vi "Corresponding Answer (SubVI).vi"(1 "Command":string, 2 "Tracker Response":string) -> (8 "Boolean":bool)   [LabVIEW 2017]
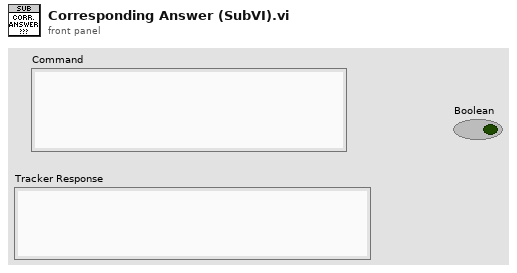
[diagram p1: front panel]
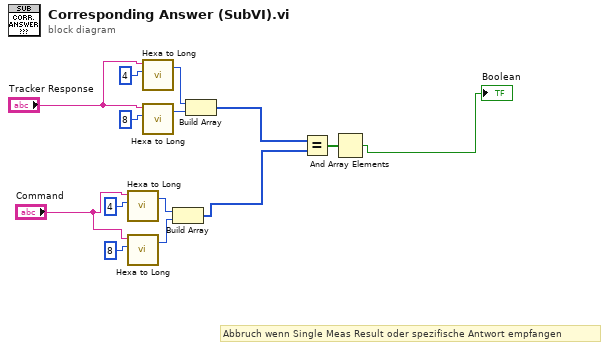
[diagram p0: block diagram]
diagram:
  # "Abbruch wenn Single Meas Result oder spezifische Antwort empfangen"
  n1 = call "Hexa to Long.vi"("Hexa"="Command", "Index"=4) -> ("Long"=w5:u32)  [unwired: 4 in]
  n2 = call "Hexa to Long.vi"("Hexa"="Command", "Index"=8) -> ("Long"=w4:u32)  [unwired: 4 in]
  n3 = call "Hexa to Long.vi"("Hexa"="Tracker Response", "Index"=4) -> ("Long"=w2:u32)  [unwired: 4 in]
  n4 = call "Hexa to Long.vi"("Hexa"="Tracker Response", "Index"=8) -> ("Long"=w9:u32)  [unwired: 4 in]
  n5 = Build Array(w5, w4) -> (w3:u32[])
  n6 = Build Array(w2, w9) -> (w12:u32[])
  n7 = Equal?(x=w12, y=w3) -> (x = y?=w13:bool[])
  n8 = And Array Elements(Boolean array=w13) -> (logical AND=→"Boolean":bool)
